vi "2021_day5_task1.vi"() -> ()   [LabVIEW 2021]
panel:
  out "Total Overlap Points":i16
  out "result string":string
  out "Array 2":i32[][](array[numeric])
  out "Array":T1(array[cluster])
  out "array":string[](array[string])
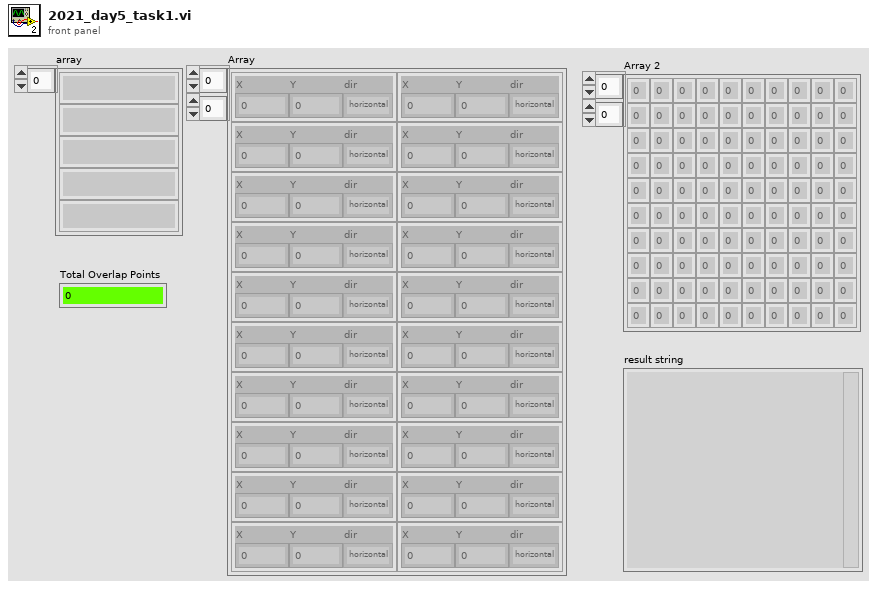
[diagram p1: front panel]
types:
  T1 = cluster{"X":i32, "Y":i32, "dir":enum16{"horizontal", "vertical"}}[][]
  T2 = cluster{"X":i32, "Y":i32, "dir":enum16{"horizontal", "vertical"}}
  T3 = cluster{"X":i32, "Y":i32, "dir":enum16{"horizontal", "vertical"}}[]
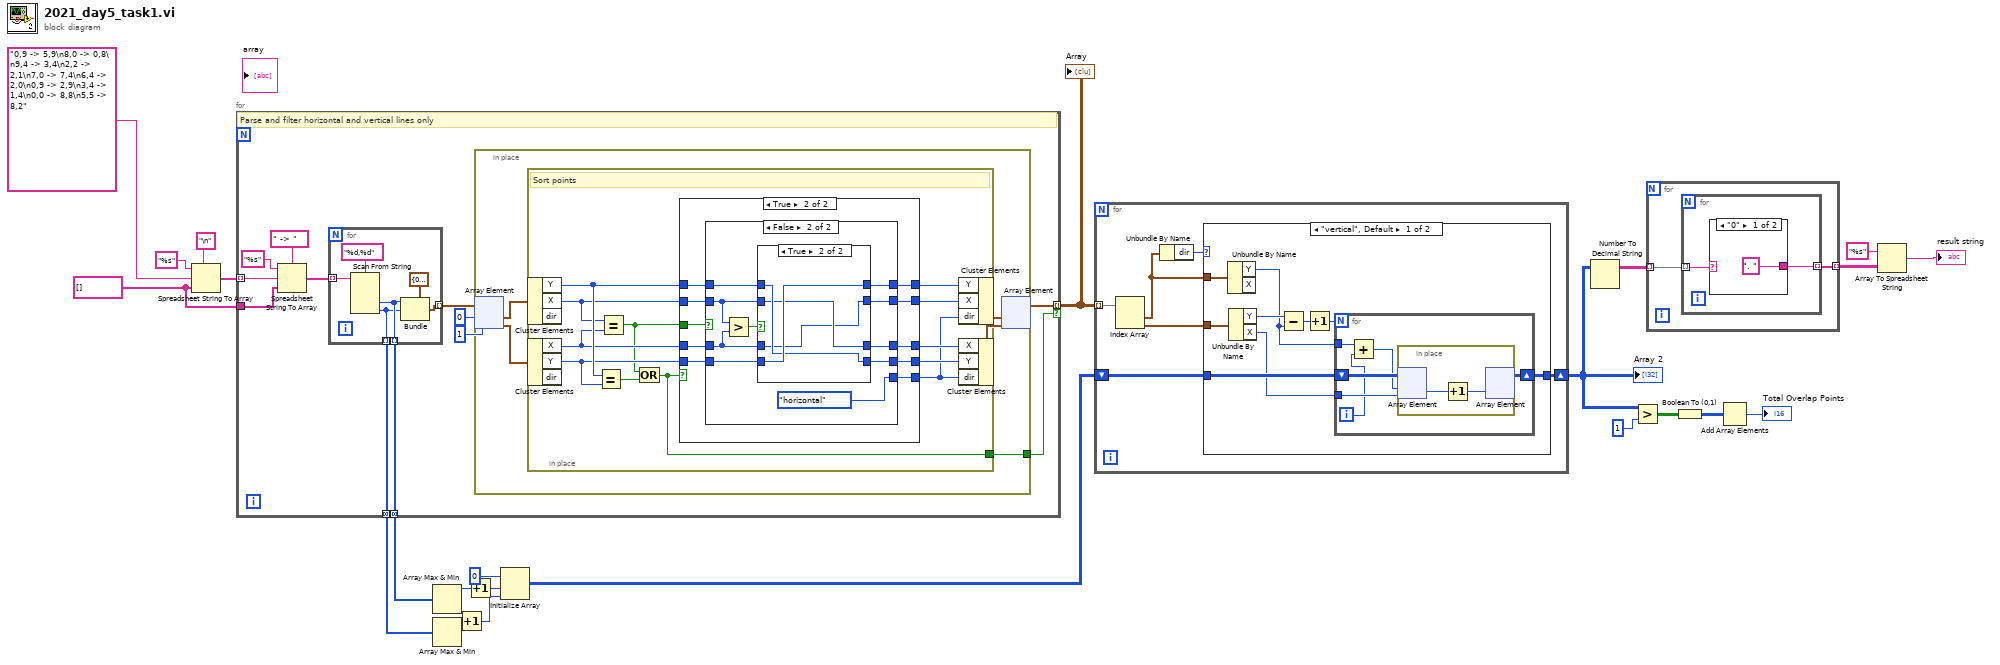
[diagram p0: block diagram]
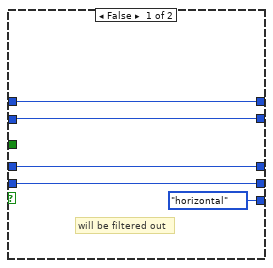
[diagram p3: hidden frame]
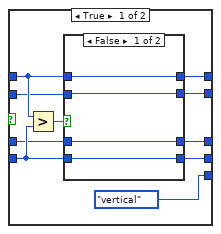
[diagram p4: hidden frame]
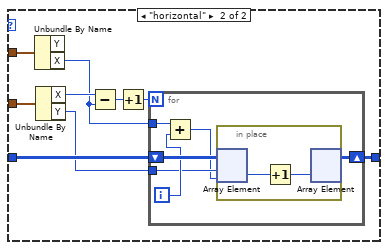
[diagram p7: hidden frame]
diagram:
  w19 = string[] [] ("array type (2D Dbl)")
  n1 = Spreadsheet String To Array(delimiter (Tab)="\n", format string="%s", spreadsheet string="0,9 -> 5,9\n8,0 -> 0,8\n9,4 -> 3,4\n2,2 -> 2,1\n7,0 -> 7,4\n6,4 -> 2,0\n0,9 -> 2,9\n3,4 -> 1,4\n0,0 -> 8,8\n5,5 -> 8,2", array type (2D Dbl)=w19) -> (array=w20:string[])
  n2 = for {
    tunnel: w20 -> [w34] mode=indexing
    tunnel: w19 -> [w32]
    tunnel: [w29] -> w18 mode=indexing if=w28
    tunnel: [w25] -> w16 mode=concatenating
    tunnel: [w24] -> w17 mode=concatenating
    # "Parse and filter horizontal and vertical lines only"
    n3 = Spreadsheet String To Array(delimiter (Tab)=" -> ", format string="%s", spreadsheet string=w34, array type (2D Dbl)=w32) -> (array=w31:string[])
    n4 = for {
      tunnel: w31 -> [w41] mode=indexing
      tunnel: [w39] -> w30 mode=indexing
      tunnel: [w37] -> w25 mode=indexing
      tunnel: [w36] -> w24 mode=indexing
      n5 = Scan From String(format string="%d,%d", input string=w41) -> (output 1=w37:i32, output 2=w36:i32)  [unwired: 4 in, 3 out]
      n6 = Bundle(cluster=T2 {"X"=0, "Y"=0, "dir"=enum."horizontal"}, "X"=w37, "Y"=w36) -> (w39:T2)  [unwired: 1 in]
    }
    n7 = in-place {
      in-place-border: [w44] -> w28
      n8 = in-place-array #1(w30, 0, 1) -> (w46:T2, w45:T2)
      n9 = in-place {
        in-place-border: [w48] -> w44
        # "Sort points"
        n10 = in-place-cluster #2(w46) -> ("Y"=w57:i32, "X"=w55:i32)  [unwired: 1 out]
        n11 = in-place-cluster #3(w45) -> ("X"=w54:i32, "Y"=w56:i32)  [unwired: 1 out]
        n12 = Equal?(x=w57, y=w56) -> (x = y?=w58:bool)
        n13 = Equal?(x=w55, y=w54) -> (x = y?=w49:bool)
        n14 = Or(x=w49, y=w58) -> (x .or. y?=w48:bool)
        n15 = case shown="True" w48 {
          tunnel: w57 -> [w63 w73]
          tunnel: w56 -> [w60 w72]
          tunnel: w55 -> [w62 w71]
          tunnel: w54 -> [w61 w70]
          tunnel: [w63 w69] -> w53
          tunnel: [w62 w68] -> w52
          tunnel: [w61 w67] -> w51
          tunnel: [w60 w66] -> w50
          tunnel: w49 -> [_ w65]
          tunnel: [enum16{"horizontal", "vertical"}."horizontal" ("dir") w64] -> w47
          frame False {
            # "will be filtered out"
          }
          frame True {
            n16 = case shown="False" w65 {
              tunnel: w73 -> [w83 w101]
              tunnel: w72 -> [w82 w100]
              tunnel: w71 -> [w80 w94]
              tunnel: w70 -> [w79 w93]
              tunnel: [w78 w98] -> w69
              tunnel: [w77 w97] -> w68
              tunnel: [w76 w96] -> w67
              tunnel: [w75 w95] -> w66
              tunnel: [enum16{"horizontal", "vertical"}."vertical" ("dir") enum16{"horizontal", "vertical"}."horizontal" ("dir")] -> w64
              frame True {
                n17 = Greater?(x=w83, y=w82) -> (0:w81:bool)
                n18 = case shown="False" w81 {
                  tunnel: w83 -> [w87 w90]
                  tunnel: w82 -> [w84 w91]
                  tunnel: w80 -> [w86 w89]
                  tunnel: w79 -> [w85 w88]
                  tunnel: [w87 w91] -> w78
                  tunnel: [w86 w88] -> w77
                  tunnel: [w85 w89] -> w76
                  tunnel: [w84 w90] -> w75
                  frame False {
                  }
                  frame True {
                  }
                }
              }
              frame False {
                n19 = Greater?(x=w94, y=w93) -> (0:w99:bool)
                n20 = case shown="True" w99 {
                  tunnel: w101 -> [w105 w108]
                  tunnel: w100 -> [w102 w109]
                  tunnel: w94 -> [w104 w107]
                  tunnel: w93 -> [w103 w106]
                  tunnel: [w105 w109] -> w98
                  tunnel: [w104 w106] -> w97
                  tunnel: [w103 w107] -> w96
                  tunnel: [w102 w108] -> w95
                  frame False {
                  }
                  frame True {
                  }
                }
              }
            }
          }
        }
        n21 = in-place-cluster #2("Y"=w53, "X"=w52, "dir"=w47) -> (w43:T2)
        n22 = in-place-cluster #3("X"=w51, "Y"=w50, "dir"=w47) -> (w42:T2)
      }
      n23 = in-place-array #1(w43, w42) -> (w29:T3)  [unwired: 2 out]
    }
  }
  "Array" <- w18
  n24 = Array Max & Min(array=w16) -> (max value=w14:i32)  [unwired: 3 out]
  n25 = Array Max & Min(array=w17) -> (max value=w13:i32)  [unwired: 3 out]
  n26 = Increment(x=w13) -> (x+1=w10:i32)
  n27 = Increment(x=w14) -> (x+1=w11:i32)
  n28 = Initialize Array(0, w11, w10) -> (w12:i32[][])
  n29 = for {
    tunnel: w18 -> [w115] mode=indexing
    shift-right: [w110] -> w1
    shift-left: w12 -> [w111]
    n30 = Index Array(array=w115) -> (element #1=w113:T2, element #2=w114:T2)  [unwired: 2 in]
    n31 = Unbundle By Name(w113) -> ("dir"=w112:enum16{"horizontal", "vertical"})
    n32 = case shown="\"vertical\", Default" w112 {
      tunnel: w114 -> [w124 w141]
      tunnel: w113 -> [w123 w140]
      tunnel: w111 -> [w122 w139]
      tunnel: [w121 w138] -> w110
      frame "vertical", Default {
        n33 = Unbundle By Name(w123) -> ("Y"=w117:i32)  [unwired: 1 out]
        n34 = Unbundle By Name(w124) -> ("Y"=w119:i32, "X"=w120:i32)
        n35 = Subtract(x=w119, y=w117) -> (x-y=w118:i32)
        n36 = Increment(x=w118) -> (x+1=w116:i32)
        n37 = for {
          N: w116 -> [_]
          shift-right: [w129] -> w121
          shift-left: w122 -> [w130]
          tunnel: w120 -> [w128]
          tunnel: w117 -> [w127]
          i -> [w126]
          n38 = Add(x=w127, y=w126) -> (x+y=w125:i32)
          n39 = in-place {
            n40 = in-place-array #4(w130, w125, w128) -> (w132:i32)
            n41 = Increment(x=w132) -> (x+1=w131:i32)
            n42 = in-place-array #4(w131) -> (w129:i32[][])  [unwired: 2 out]
          }
        }
      }
      frame "horizontal" {
        n43 = Unbundle By Name(w140) -> ("X"=w133:i32)  [unwired: 1 out]
        n44 = Unbundle By Name(w141) -> ("X"=w136:i32, "Y"=w137:i32)
        n45 = Subtract(x=w136, y=w133) -> (x-y=w135:i32)
        n46 = Increment(x=w135) -> (x+1=w134:i32)
        n47 = for {
          N: w134 -> [_]
          shift-right: [w146] -> w138
          shift-left: w139 -> [w147]
          tunnel: w137 -> [w143]
          tunnel: w133 -> [w145]
          i -> [w144]
          n48 = Add(x=w145, y=w144) -> (x+y=w142:i32)
          n49 = in-place {
            n50 = in-place-array #5(w147, w143, w142) -> (w149:i32)
            n51 = Increment(x=w149) -> (x+1=w148:i32)
            n52 = in-place-array #5(w148) -> (w146:i32[][])  [unwired: 2 out]
          }
        }
      }
    }
  }
  "Array 2" <- w1
  n53 = Number To Decimal String(number=w1) -> (decimal integer string=w9:string[][])  [unwired: 1 in]
  n54 = Greater?(x=w1, y=1) -> (0:w4:bool[][])
  n55 = for {
    tunnel: w9 -> [w151] mode=indexing
    tunnel: [w150] -> w8 mode=indexing
    n56 = for {
      tunnel: w151 -> [w153] mode=indexing
      tunnel: [w152] -> w150 mode=indexing
      n57 = case shown="\"0\"" w153 {
        selector: w153 -> [_ w155]
        tunnel: [". " ("replace string (\"\")") w155] -> w152
        frame "0" {
        }
        frame "1", Default {
        }
      }
    }
  }
  n58 = Boolean To (0,1)(Boolean=w4) -> (0, 1=w3:i16[][])
  n59 = Add Array Elements(numeric array=w3) -> (sum=→"Total Overlap Points":i16)
  n60 = Array To Spreadsheet String(array=w8, 3:"%s" ("format string")) -> (spreadsheet string=→"result string":string)  [unwired: 1 in]
